vi "EMD8216 subnet mask read.vi"(11 "CardID":u32) -> (1 "subnet_mask":u8[](array[numeric]), 3 "error_code":u32)   [LabVIEW 2009, in "EMD8216_64.lvlib"]
doc: "EMD8216Status EMD8216_subnet_mask_read(u32 CardID,u8 subnet_mask[4]);"
uses:
  EMD8216_64.lvlib
  <userlib>/EMD8216_64/EMD8216_64.dll
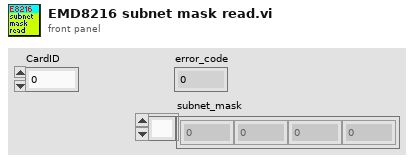
[diagram p1: front panel]
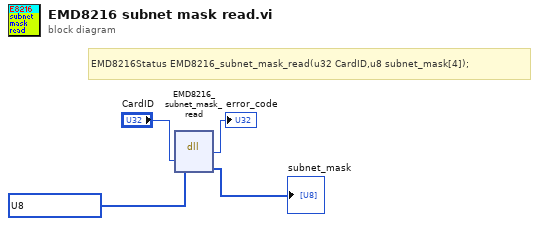
[diagram p0: block diagram]
diagram:
  # "EMD8216Status EMD8216_subnet_mask_read(u32 CardID,u8 subnet_mask[4]);"
  n1 = dll-call lib="C:/Program Files/National Instruments/LabVIEW 2017/user.lib/EMD8216_64/EMD8216_64.*" fn="EMD8216_subnet_mask_read"("CardID"="CardID", "subnet_mask"=u8[] ?) -> ("return type"=→"error_code":u32, "subnet_mask"=→"subnet_mask":u8[])  [unwired: 4 in, 2 out]
